vi "RT Train PID_RIO.vi"() -> ()   [LabVIEW 2018]
uses:
  <vilib>/myRIO/Instrument Drivers/Onboard IO/AO/typedefs/AO Reference.ctl
  <vilib>/myRIO/Common/Instrument Driver Framework/Utilities/typedefs/myRIO Generic Hardware Reference.ctl
  <vilib>/myRIO/Common/Instrument Driver Framework/Utilities/typedefs/Hardware Version Enum.ctl
  <vilib>/myRIO/Common/Instrument Driver Framework/Utilities/typedefs/myRIO v1.0 Reference.ctl
  <vilib>/myRIO/Common/Instrument Driver Framework/Utilities/typedefs/Generic FPGA Reference.ctl
  <vilib>/myRIO/Common/Instrument Driver Framework/myRIO v1.0/AO/typedefs/AO Channels List.ctl
  <vilib>/myRIO/Common/Instrument Driver Framework/myRIO v1.0/AO/typedefs/AO Channels Enum.ctl
  <vilib>/myRIO/Common/Instrument Driver Framework/Utilities/typedefs/Analog Scaling Constants List.ctl
  <vilib>/myRIO/Common/Instrument Driver Framework/Utilities/typedefs/Analog Scaling Constants.ctl
  <vilib>/userdefined/High Color/nirio_resource_hc.ctl
  <vilib>/Platform/TimedLoop/XDataNode/timing_clust.ctl
  <vilib>/Platform/TimedLoop/XDataNode/nitl_modes.ctl
  <vilib>/Platform/TimedLoop/XDataNode/wakeup.ctl
  <vilib>/myRIO/Common/Instrument Driver Framework/Utilities/vis/Is FPGA Ref Available.vi
  <vilib>/myRIO/Common/Instrument Driver Framework/myRIO v1.0/AO/vis/myRIO v1.1 Open AO.vi
  <vilib>/myRIO/Instrument Drivers/Onboard IO/AO/vis/Write.vi
  <vilib>/myRIO/Common/Instrument Driver Framework/Utilities/vis/Validate Channels.vi
  <vilib>/myRIO/Common/Instrument Driver Framework/myRIO v1.0/AO/vis/myRIO v1.0 Reserve AO.vi
  <vilib>/myRIO/Common/Instrument Driver Framework/myRIO v1.0/AO/vis/myRIO v1.0 Build MUX Configuration AO.vi
  <vilib>/myRIO/Common/Instrument Driver Framework/myRIO v1.0/Resource Manager/vis/myRIO v1.0 Reserve Channel List.vi
  <vilib>/myRIO/Common/Instrument Driver Framework/myRIO v1.0/Resource Manager/vis/myRIO v1.0 Reserve Channel.vi
  <vilib>/myRIO/Common/Instrument Driver Framework/myRIO v1.0/Resource Manager/vis/myRIO v1.0 Unreserve Channel.vi
  <vilib>/myRIO/Common/Instrument Driver Framework/myRIO v1.0/Resource Manager/vis/myRIO v1.0 Build Mutex Name.vi
  <vilib>/Utility/VariantDataType/GetNumericInfo.vi
  <vilib>/Utility/error.llb/Error Cluster From Error Code.vi
  <vilib>/myRIO/Common/Instrument Driver Framework/myRIO v1.0/myRIO v1.1 Open.vi
  <vilib>/myRIO/Common/Instrument Driver Framework/myRIO v1.0/AO/vis/myRIO v1.0 Get Scaling Constants AO.vi
  <vilib>/myRIO/Common/Instrument Driver Framework/Utilities/vis/IO Manager.vi
  <vilib>/myRIO/Common/Instrument Driver Framework/Utilities/vis/Configuration Manager.vi
  <vilib>/myRIO/Common/Instrument Driver Framework/myRIO v1.0/myRIO v1.0 Close.vi
  <vilib>/myRIO/Common/Instrument Driver Framework/myRIO v1.0/AO/vis/myRIO v1.0 Write AO.vi
  <vilib>/addons/control/pid/pid.llb/PID (DBL).vi
  <vilib>/myRIO/Express VI/Onboard IO/AO/AO Express VI.xnode
  <vilib>/myRIO/Instrument Drivers/Onboard IO/AO/vis/myRIO AO Open.xnode
  <vilib>/platform/TimedLoop/XDataNode/XDataNode.xnode
  <vilib>/addons/control/pid/NI_PID_pid.lvlib
  <vilib>/myRIO/Instrument Drivers/Onboard IO/AO/AO.lvlib
  <vilib>/Platform/TimedLoop/XDataNode/XDNodeRunTimeDep.lvlib
panel:
  in  "stop":bool
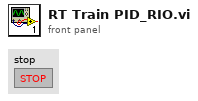
[diagram p1: front panel]
types:
  T1 = typedef "AO.lvlib/AO Reference.ctl" = cluster{"myRIO Reference":T2, "AO Channel List":T6, "AO Scaling Constant List":T8}
  T2 = typedef "myRIO Generic Hardware Reference.ctl" = cluster{"myRIO Model":T3, "myRIO Hardware Reference":T4}
  T3 = typedef "Hardware Version Enum.ctl" = enum16{"Unknown", "myRIO-1900", "myRIO-1950", "roboRIO", "NI ELVIS RIO CM", "ELVIS III"}
  T4 = typedef "myRIO v1.0 Reference.ctl" = cluster{"Generic FPGA Reference":T5, "Allow multiple opens":bool}
  T5 = typedef "Generic FPGA Reference.ctl" = refnum<k20>
  T6 = typedef "AO Channels List.ctl" = T7[]
  T7 = typedef "AO Channels Enum.ctl" = enum16{"Not Connected", "AudioOut/Left", "AudioOut/Right", "C/AO0", "C/AO1", "A/AO0", "A/AO1", "B/AO0", "B/AO1"}
  T8 = typedef "Analog Scaling Constants List.ctl" = T9[]
  T9 = typedef "Analog Scaling Constants.ctl" = cluster{"LSB Weight (Volts)":dbl, "Offset (Volts)":dbl, "Signed?":bool}
  T10 = typedef "nirio_resource_hc.ctl" = tag
  T11 = typedef "XDNodeRunTimeDep.lvlib/timing_clust.ctl" = cluster{"Expected End [f-1]":u64, "Actual End [f-1]":u64, "Finished Late? [f-1]":bool, "Expected End [i-1]":u64, "Actual End [i-1]":u64, "Finished Late? [i-1]":bool, "Expected Start [i]":u64, "Actual Start [i]":u64, "Expected Start [f]":u64, "Actual Start [f]":u64, "Source Name":string, "Structure Name":string, "Period":i64, "Deadline":i64, "Offset":i64, "Start":i64, "Priority":i32, "Timeout":i32, "Mode":T12, "Wakeup Reason":T13, "Error":errorcluster, "Source Type":string, "Secondary Source Type":string, "Global End Time":u64, "Global Start Time":u64, "Frame Duration":u64, "Iteration Duration":u64, "Assigned CPU":i32, "I/O Scan Engine Mode":u32}
  T12 = typedef "XDNodeRunTimeDep.lvlib/nitl_modes.ctl" = enum32{"No Change", "Process missed periods, maintain original phase", "Discard missed periods, maintain original phase", "Process missed periods, ignore original phase", "Discard missed periods, ignore original phase"}
  T13 = typedef "XDNodeRunTimeDep.lvlib/wakeup.ctl" = enum32{"Normal", "Aborted", "Asynchronous wakeup", "Timing source error", "Timed loop error", "Timeout"}
  T14 = cluster{"proportional gain (Kc)":dbl, "integral time (Ti, min)":dbl, "derivative time (Td, min)":dbl}
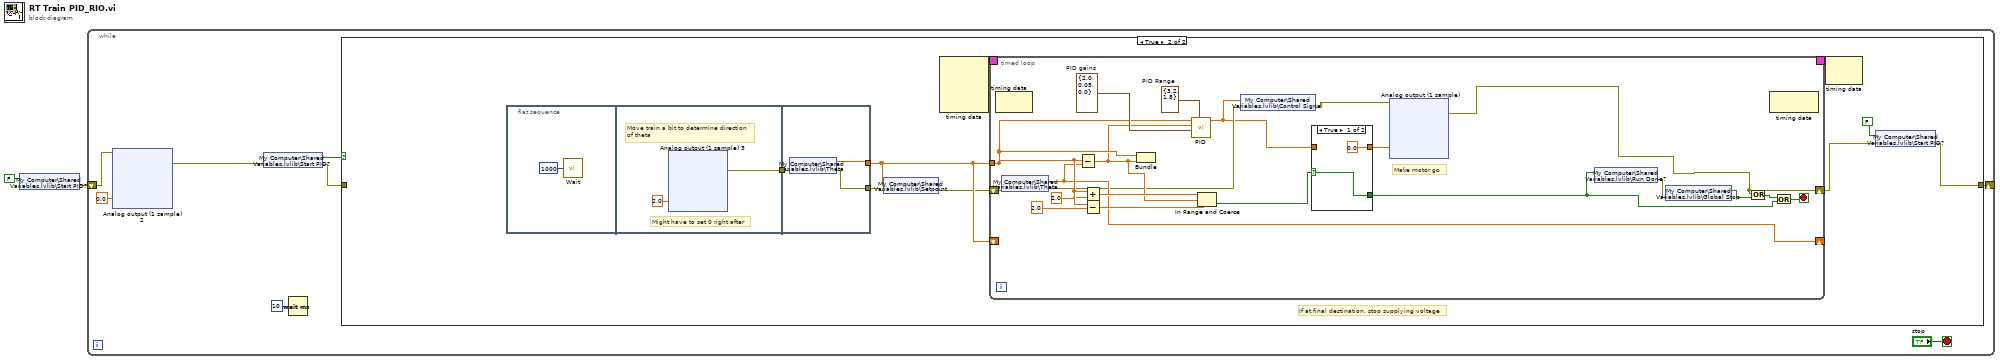
[diagram p0: block diagram]
diagram:
  n1 = shared-variable "My Computer\\Shared Variables.lvlib\\Start PID?"(FALSE ("Start PID?")) -> (error out=w1:errorcluster)  [unwired: 1 in]
  n2 = while {
    shift-right: [w4] -> _
    shift-left: w1 -> [w3]
    stop <- "stop" stop-if-true
    n3 = xnode "Analog output (1 sample) 2"("C/AO0 (AO0)"=0.0, "error in (no error)"=w3) -> ("error out"=w6:errorcluster)
    n4 = shared-variable "My Computer\\Shared Variables.lvlib\\Start PID?"(error in=w6) -> (w9:bool, error out=w5:errorcluster)
    n5 = Wait (ms)(milliseconds to wait=u32 10) -> ()  [unwired: 1 out]
    n6 = case shown="True" w9 {
      tunnel: w5 -> [w48 _]
      tunnel: [w48 w49] -> w4
      frame False {
      }
      frame True {
        # "If at final destination, stop supplying voltage"
        n7 = flat-sequence {
          tunnel: [w59] -> w55
          tunnel: [w100] -> w51
          tunnel: [w99] -> w54
          tunnel: w55 -> [w98]
          frame #0 {
            n8 = call "Wait"("Count(mSec)"=u32 1000) -> ()  [unwired: 1 out]
          }
          frame #1 {
            # "Might have to set 0 right after"
            # "Move train a bit to determine direction\nof theta"
            n9 = xnode "Analog output (1 sample) 3"("C/AO0 (AO0)"=2.0) -> ("error out"=w59:errorcluster)  [unwired: 1 in]
          }
          frame #2 {
            n10 = shared-variable "My Computer\\Shared Variables.lvlib\\Theta"(error in=w98) -> (w100:dbl, error out=w99:errorcluster)
          }
        }
        n11 = shared-variable "My Computer\\Shared Variables.lvlib\\Setpoint"(w51, error in=w54) -> (error out=w50:errorcluster)
        n12 = node-c288() -> (w57:T11)  [unwired: 4 in]
        n13 = timed-loop {
          timing: w57 -> [_]
          timing-out: [_] -> w56
          tunnel: w51 -> [w119]
          shift-right: [w106] -> _
          shift-left: w51 -> [_]
          shift-right: [w101] -> w53
          shift-left: w50 -> [w105]
          stop <- w111 stop-if-true
          w120 = T14 {"proportional gain (Kc)"=2.0, "integral time (Ti, min)"=0.05, "derivative time (Td, min)"=0.0}  # PID gains
          w121 = cluster{"output high":dbl, "output low":dbl} {"output high"=3.2, "output low"=1.8}  # PID Range
          # "Make motor go"
          n14 = node-c288() -> ()  [unwired: 1 in, 1 out]
          n15 = shared-variable "My Computer\\Shared Variables.lvlib\\Theta"(error in=w105) -> (w106:dbl, error out=w104:errorcluster)
          n16 = Subtract(x=w119, y=w106) -> (x-y=w107:dbl)
          n17 = Add(x=w119, y=2.0) -> (x+y=w116:dbl)
          n18 = Subtract(x=w119, y=2.0) -> (x-y=w115:dbl)
          n19 = Bundle("Double"=w119, w107) -> ()  [unwired: 1 in, 1 out]
          n20 = call-poly <vilib>:"PID.vi"("output range"=w121, "PID gains"=w120, "process variable"=w107, "setpoint"=w119) -> ("output"=w102:dbl)  [unwired: 6 in, 1 out]
          n21 = In Range and Coerce(upper limit=w116, x=w107, lower limit=w115) -> (In Range?=w114:bool)  [unwired: 1 out]
          n22 = shared-variable "My Computer\\Shared Variables.lvlib\\Control Signal"(w102, error in=w104) -> (error out=w103:errorcluster)
          n23 = case shown="True" w114 {
            selector: w114 -> [w122 w124]
            tunnel: [0.0 ("output") w125] -> w113
            tunnel: w102 -> [_ w125]
            tunnel: [w122 w124] -> w109
            frame True {
            }
            frame False {
            }
          }
          n24 = xnode "Analog output (1 sample)"("C/AO0 (AO0)"=w113, "error in (no error)"=w103) -> ("error out"=w101:errorcluster)
          n25 = shared-variable "My Computer\\Shared Variables.lvlib\\Run Done?"(w109) -> (error out=w108:errorcluster)  [unwired: 1 in]
          n26 = shared-variable "My Computer\\Shared Variables.lvlib\\Global Stop"(error in=w108) -> (w112:bool)  [unwired: 1 out]
          n27 = Or(x=w101, y=w112) -> (x .or. y?=w110:bool)
          n28 = node-c288() -> ()  [unwired: 1 in, 1 out]
          n29 = Or(x=w110, y=w109) -> (x .or. y?=w111:bool)
        }
        n30 = node-c288(w56) -> ()  [unwired: 1 out]
        n31 = shared-variable "My Computer\\Shared Variables.lvlib\\Start PID?"(FALSE ("Start PID?"), error in=w53) -> (error out=w49:errorcluster)
      }
    }
  }
